vi "CalWaypoint.vi"(7 "InhibitIn":bool, 8 "CurrentSteerAngle":dbl, 9 "WhereAmI?":T3, 11 "MDD In":T4[](array[typedef])) -> (0 "Forebrain Command":T1, 1 "MDF Out":T4[](array[typedef]), 2 "ActCommand":dbl[](array[numeric]), 3 "Current State":i32, 4 "InhibitOut":bool, 5 "Vel":dbl, 6 "SteerAngle":dbl)   [LabVIEW 2011]
doc: "This subVI contains the Forebrain Goto Waypoint behaviors. Its inputs are the outputs of thewhat and where SENSE processes, theMission efinition Filet, a suppression value from another co-brahvior and an inhibit signal to turn the behavior off. The outputs are a 90 element steering array and a suppression value to diminish the output of co-behaviors.\n\nIt is designed to work with a 90 element behavior arbiter."
uses:
  MDF.ctl
  Behaviour.ctl
  WhereAmI.ctl
  ForebrainCmd.ctl
  <vilib>/Analysis/1siggen.llb/Ramp Pattern by Samples.vi
  <vilib>/gmath/statdist.llb/Normal PDF.vi
  <vilib>/gmath/NI_Gmath.lvlib
  <vilib>/Analysis/NI_AALBase.lvlib
panel:
  out "Old MDF Out":T5(array[cluster])
  out "loop index":i32
  # "This VI contains the go to waypoint behavior  at the Forebrain level"
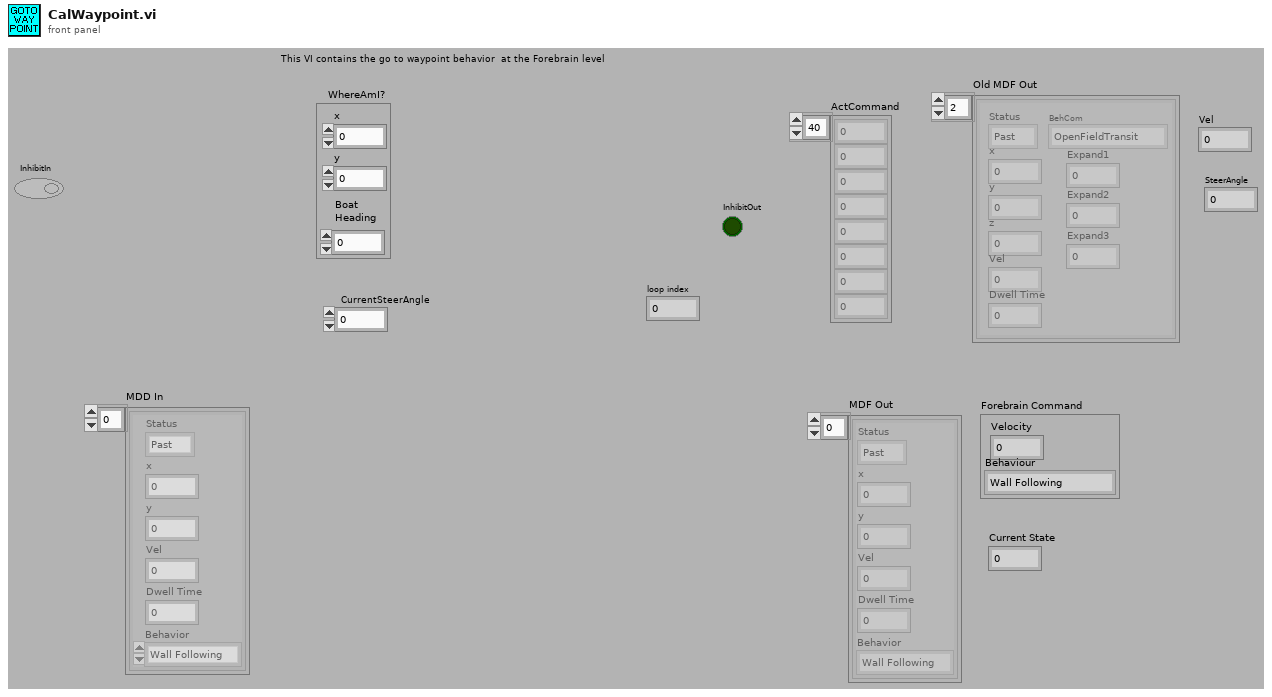
[diagram p1: front panel]
types:
  T1 = typedef "ForebrainCmd.ctl" = cluster{"Velocity":dbl, "Behaviour":T2}
  T2 = typedef "Behaviour.ctl" = enum16{"Wall Following", "Open Transit", "Find Barge", "Push Barge", "Go Home"}
  T3 = typedef "WhereAmI.ctl" = cluster{"x":sgl, "y":sgl, "Boat\nHeading":sgl}
  T4 = typedef "MDF.ctl" = cluster{"Status":enum16{"Past", "Current", "Future"}, "x":dbl, "y":dbl, "Vel":dbl, "Dwell Time":dbl, "Behavior":T2}
  T5 = cluster{"Status":enum16{"Past", "Current", "Future"}, "x":dbl, "y":dbl, "z":dbl, "Vel":dbl, "Dwell Time":dbl, "BehCom":enum16{"OpenFieldTransit", "P-WallFollow", "S-WallFollow", "LaneFollow", "ManualMode"}, "Expand1":dbl, "Expand2":dbl, "Expand3":dbl}[]
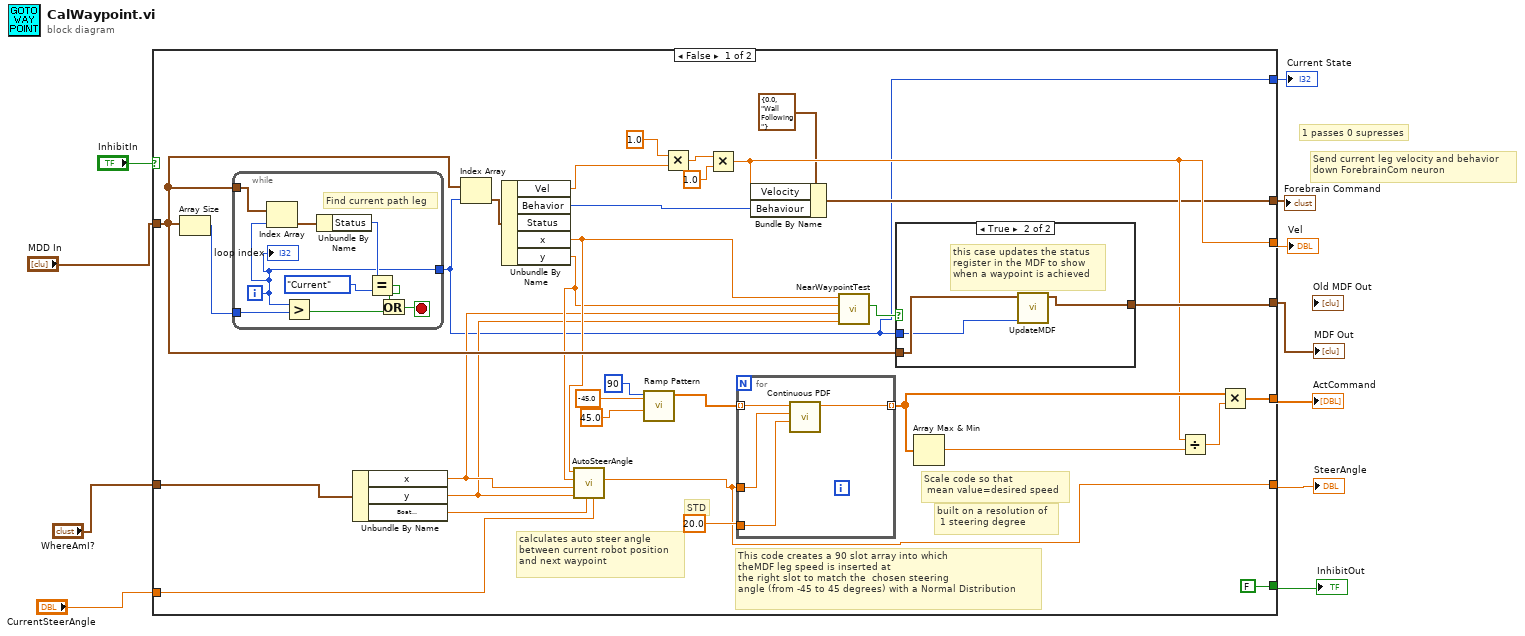
[diagram p0: block diagram]
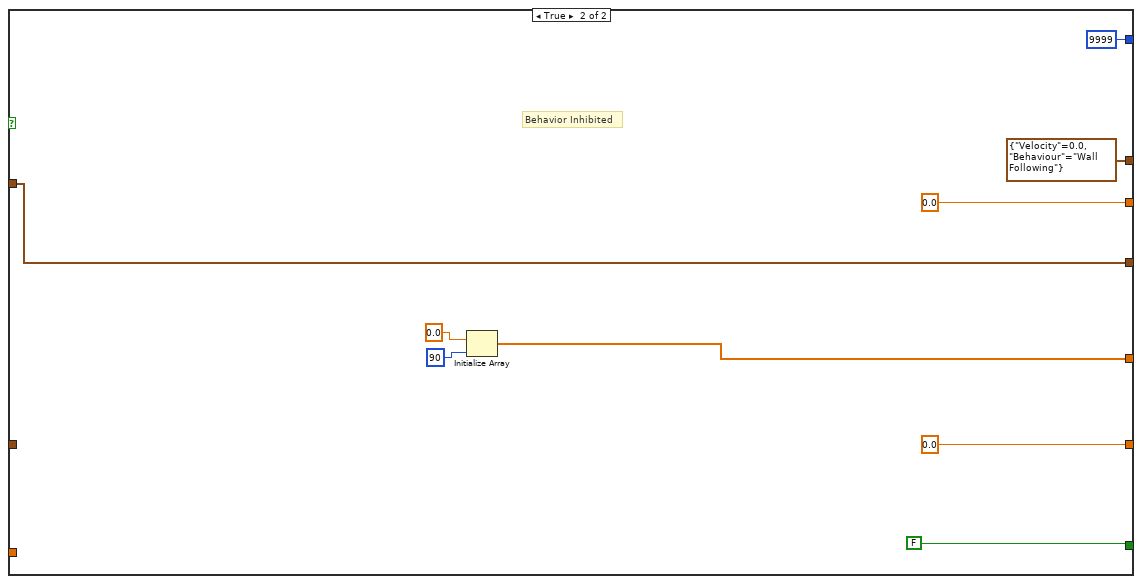
[diagram p3: hidden frame]
diagram:
  # "Send current leg velocity and behavior\ndown ForebrainCom neuron"
  # "1 passes 0 supresses"
  n1 = case shown="False" "InhibitIn" {
    tunnel: "WhereAmI?" -> [w41 _]
    tunnel: [w30 w68] -> w9
    tunnel: [FALSE ("InhibitOut") FALSE ("InhibitOut")] -> w10
    tunnel: "MDD In" -> [w27 w65]
    tunnel: [w26 w65] -> w4
    tunnel: [w17 0.0 ("Vel")] -> w8
    tunnel: [w24 0.0 ("SteerAngle")] -> w7
    tunnel: "CurrentSteerAngle" -> [w23 _]
    tunnel: [w14 T1 {"Velocity"=0.0, "Behaviour"=enum."Wall Following"} ("Forebrain Cmd")] -> w2
    tunnel: [w13 9999] -> w1
    frame False {
      # "calculates auto steer angle\nbetween current robot position\nand next waypoint"
      # "built on a resolution of\n 1 steering degree"
      # "Scale code so that\n mean value=desired speed"
      # "STD"
      # "This code creates a 90 slot array into which\ntheMDF leg speed is inserted at\nthe right slot to match the  chosen steering\nangle (from -45 to 45 degrees) with a Normal Distribution"
      n2 = Array Size(array=w27) -> (size(s)=w42:i32)
      n3 = while {
        tunnel: w42 -> [w60]
        tunnel: w27 -> [w57]
        tunnel: [w52] -> w13
        i -> [w52]
        stop <- w59 stop-if-true
        # "Find current path leg"
        n4 = Index Array "Index Array"(array=w57, index=w52) -> (element=w54:T4)
        n5 = Greater?(x=w52, y=w60) -> (0:w58:bool)
        n6 = Unbundle By Name(w54) -> ("Status"=w55:enum16{"Past", "Current", "Future"})
        n7 = Equal?(x=w55, y=enum16{"Past", "Current", "Future"}."Current") -> (x = y?=w56:bool)
        n8 = Or(x=w56, y=w58) -> (x .or. y?=w59:bool)
        "loop index" <- w52
      }
      n9 = Unbundle By Name(w41) -> ("x"=w20:sgl, "y"=w19:sgl, "Boat\nHeading"=w29:sgl)
      n10 = Index Array "Index Array"(array=w27, index=w13) -> (element=w40:T4)
      n11 = Unbundle By Name(w40) -> ("Vel"=w25:dbl, "Behavior"=w39:T2, "x"=w22:dbl, "y"=w21:dbl)  [unwired: 1 out]
      n12 = call "AutoSteerAngle.vi"("CurrentSteerAngle"=w23, "CurrentDirection"=w29, "Ycurrent"=w19, "Xcurrent"=w20, "Ywaypoint"=w21, "Xwaypoint"=w22) -> ("NewSteerAngle"=w24:dbl)  [unwired: 5 in]
      n13 = call-poly <vilib>:"Ramp Pattern.vi"("start"=45.0, "end"=-45.0 ("end (Normal)"), "samples"=90) -> ("Ramp Pattern"=w33:dbl[])  [unwired: 7 in, 1 out]
      n14 = Multiply(x=1.0, y=w25) -> (x*y=w18:dbl)
      n15 = Multiply(x=w18, y=1.0) -> (x*y=w17:dbl)
      n16 = for {
        tunnel: w33 -> [w51] mode=indexing
        tunnel: 20.0 ("std (Normal)") -> [w50]
        tunnel: [w49] -> w37 mode=indexing
        tunnel: w24 -> [w48]
        n17 = call-poly <vilib>:"Continuous PDF.vi"("std"=w50, "mean"=w48, "x"=w51) -> ("pdf(x)"=w49:dbl)  [unwired: 7 in, 1 out]
      }
      n18 = Bundle By Name(cluster=T1 {"Velocity"=0.0, "Behaviour"=enum."Wall Following"} ("Forebrain Cmd"), "Velocity"=w17, "Behaviour"=w39) -> (w14:T1)
      n19 = call "NearWaypointTest.vi"("Yrobot"=w19, "Xrobot"=w20, "Ywaypoint"=w21, "Xwaypoiny"=w22) -> ("AtWaypoint"=w28:bool)  [unwired: 7 in]
      n20 = case shown="True" w28 {
        tunnel: w27 -> [w44 w47]
        tunnel: [w44 w45] -> w26
        tunnel: w13 -> [_ w46]
        frame False {
          # "robot not near waypoint\npass MDF through unaltered"
        }
        frame True {
          # "this case updates the status\nregister in the MDF to show \nwhen a waypoint is achieved"
          n21 = call "UpdateMDF.vi"("Index"=w46, "MDF In"=w47) -> ("MDF Out"=w45:T4[])  [unwired: 9 in]
        }
      }
      n22 = Array Max & Min(array=w37) -> (max value=w35:dbl)  [unwired: 3 out]
      n23 = Divide(x=w17, y=w35) -> (x/y=w36:dbl)
      n24 = Multiply(x=w37, y=w36) -> (x*y=w30:dbl[])
    }
    frame True {
      # "Behavior Inhibited"
      n25 = Initialize Array "Initialize Array"(0.0 ("element"), 90 ("dimension size")) -> (w68:dbl[])
    }
  }
  "ActCommand" <- w9
  "InhibitOut" <- w10
  "Vel" <- w8
  "SteerAngle" <- w7
  "MDF Out" <- w4
  "Forebrain Command" <- w2
  "Current State" <- w1
